vi "PR_Update_screw_result .vi"(8 "error in (no error)":errorcluster, 10 "barcode":string="981321652", 11 "DBlink":string="Driver={ODBC Driver 17 for SQL Server};Server=localhost\\SQLEXPRESS;Database=ZDX201;UID=labview;PWD=Dsa@54137926") -> (0 "error out":errorcluster)   [LabVIEW 2019]
uses:
  <vilib>/addons/database/Connection.llb/DB Tools Open Connec (String).vi
  <vilib>/addons/database/NI_Database_API.lvlib
panel:
  out "concatenated string":string="WHERE [barcode]='321' and [position]='A' and COALESCE(h1_R, h1_T, h2_R, h2_T, h3_R, h3_T, h4_R, h4_T, h5_R, h5_T, h6_R, h6_T) is not null"
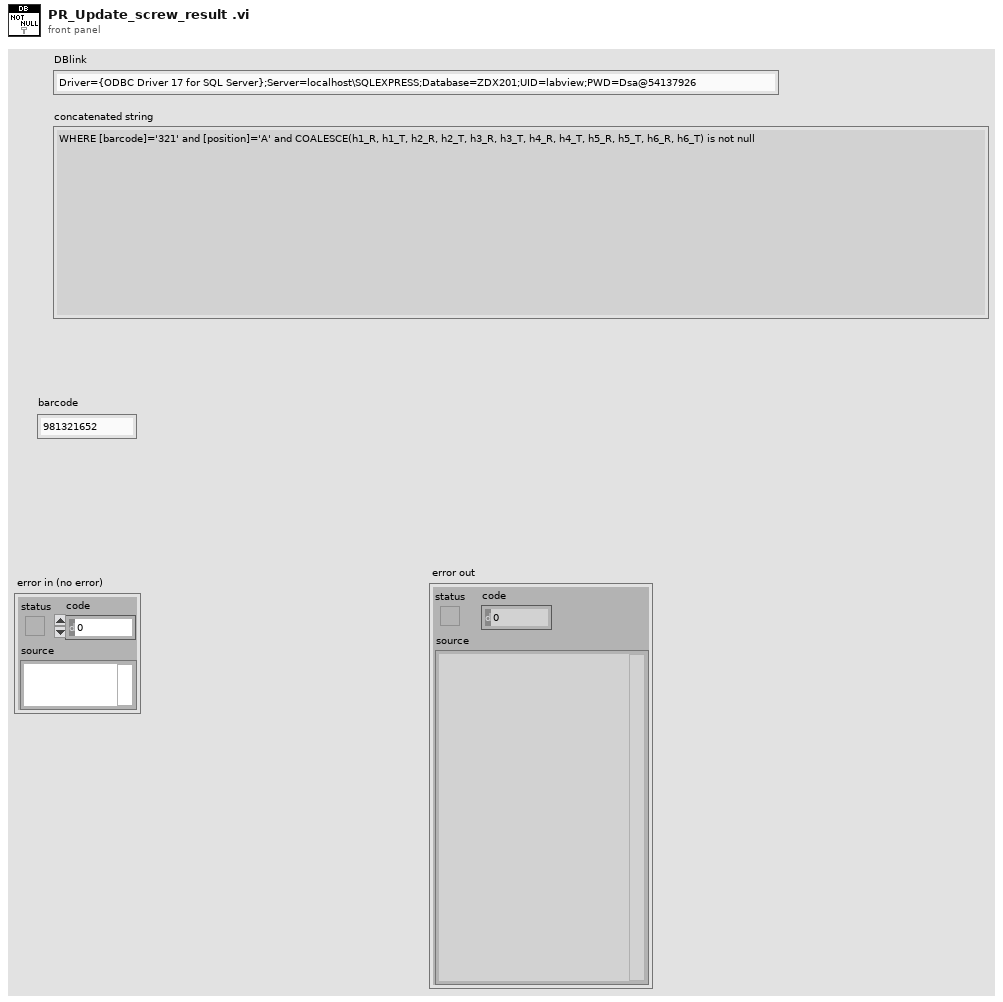
[diagram p1: front panel]
types:
  T1 = cluster{"done_time2":timestamp, "update_time":timestamp}
  T2 = typedef "NI_Database_API.lvlib/Conn ObjectReference.ctl" = refnum<k1>
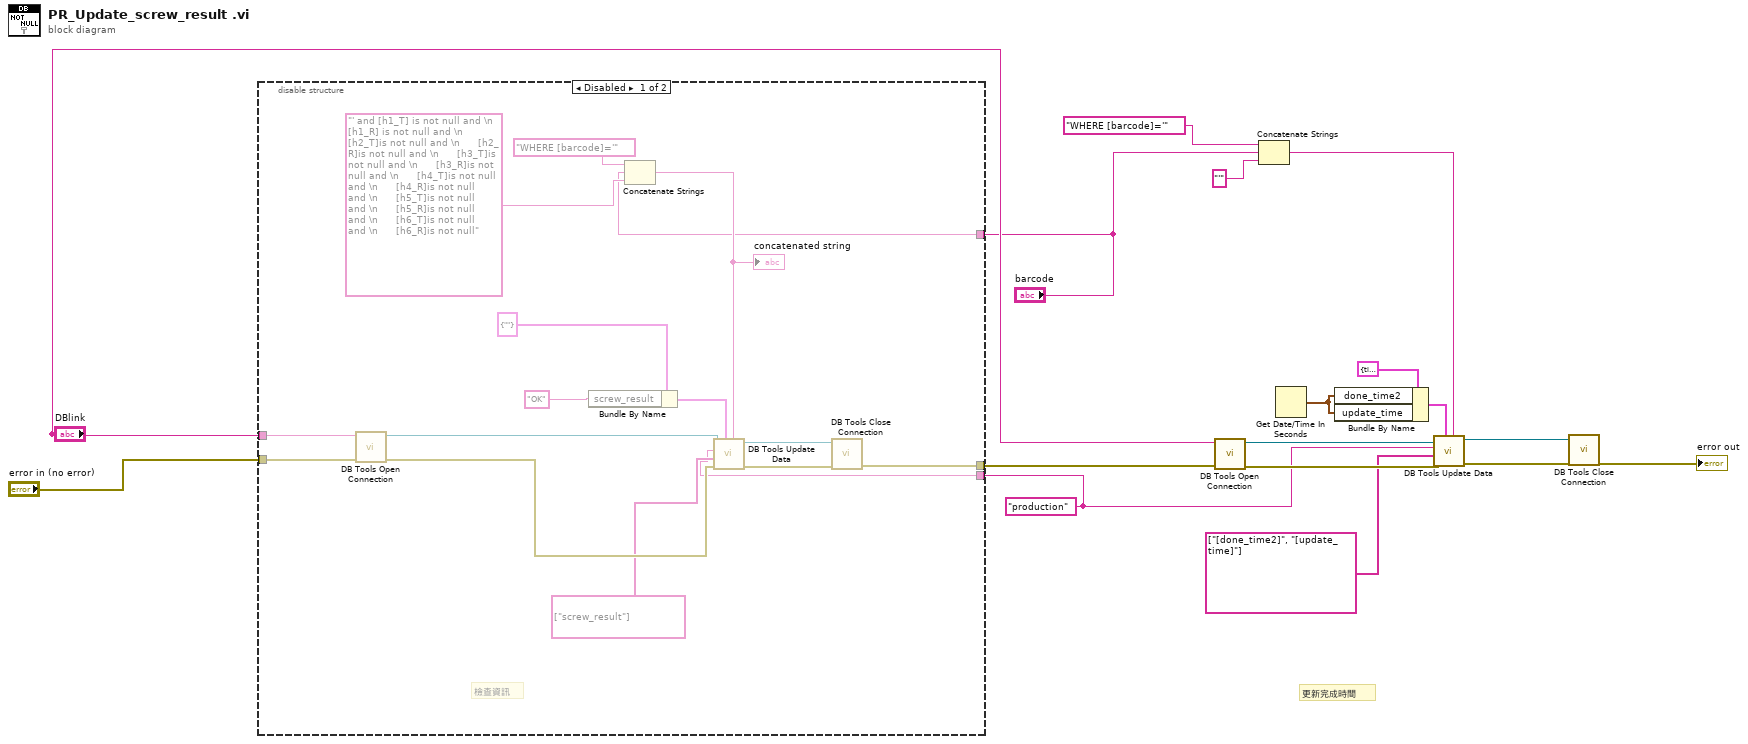
[diagram p0: block diagram]
diagram:
  w2 = "production" ("table")
  # "更新完成時間"
  n1 = disable-structure shown="Disabled" {
    disable-tunnel: "error in (no error)" -> [w32 _]
    disable-tunnel: [w20 _] -> w15
    disable-tunnel: "DBlink" -> [w19 _]
    disable-tunnel: w2 -> [w18 _]
    disable-tunnel: "barcode" -> [w17 _]
    frame Disabled {
      # "檢查資訊"
      n2 = call-poly <vilib>:"DB Tools Open Connection.vi"("error in (no error)"=w32, "connection information"=w19) -> ("error out"=w30:errorcluster, "connection reference"=w28:T2)  [unwired: 6 in]
      n3 = Bundle By Name(cluster=cluster{"screw_result":string} {"screw_result"=""}, "screw_result"="OK") -> (w22:cluster{"screw_result":string})
      n4 = Concatenate Strings("WHERE [barcode]='", w17, "' and [h1_T] is not null and \n      [h1_R] is not null and \n      [h2_T]is not null and \n      [h2_R]is not null and \n      [h3_T]is not null and \n      [h3_R]is not null and \n      [h4_T]is not null and \n      [h4_R]is not null and \n      [h5_T]is not null and \n      [h5_R]is not null and \n      [h6_T]is not null and \n      [h6_R]is not null" ("string")) -> (w25:string)
      "concatenated string" <- w25
      n5 = call <vilib>:"DB Tools Update Data.vi"("condition"=w25, "data"=w22, "error in (no error)"=w30, "columns"=string[] ["screw_result"], "table"=w18, "connection reference"=w28) -> ("error out"=w31:errorcluster, "connection reference out"=w29:T2)  [unwired: 4 in]
      n6 = call <vilib>:"DB Tools Close Connection.vi"("error in (no error)"=w31, "connection reference"=w29) -> ("error out"=w20:errorcluster)  [unwired: 5 in]
    }
    frame Enabled {
    }
  }
  n7 = call-poly <vilib>:"DB Tools Open Connection.vi"("error in (no error)"=w15, "connection information"="DBlink") -> ("error out"=w10:errorcluster, "connection reference"=w3:T2)  [unwired: 6 in]
  n8 = Concatenate Strings("WHERE [barcode]='", "barcode", "'" ("string")) -> (w6:string)
  n9 = Get Date/Time In Seconds() -> (seconds since 1Jan1904=w11:timestamp)
  n10 = Bundle By Name(cluster=T1 {"done_time2"=timestamp(0 s since 1904-01-01), "update_time"=timestamp(0 s since 1904-01-01)} ("input cluster"), "done_time2"=w11, "update_time"=w11) -> (w13:T1)
  n11 = call <vilib>:"DB Tools Update Data.vi"("condition"=w6, "data"=w13, "error in (no error)"=w10, "columns"=string[] ["[done_time2]", "[update_time]"], "table"=w2, "connection reference"=w3) -> ("error out"=→"error out":errorcluster, "connection reference out"=w4:T2)  [unwired: 4 in]
  n12 = call <vilib>:"DB Tools Close Connection.vi"("connection reference"=w4) -> ()  [unwired: 6 in, 1 out]
